vi "LVObject to JSON - No Data Member - Returns Type.vi"() -> ()   [LabVIEW 2017, in "Generic Object Serializer Tests.lvlib" / "Type Name Handling.lvlib"]
uses:
  Type Name Handling.lvlib
  No Data Member Subclass/No Data Member Subclass.lvclass
  Generic Object Serializer/Generic Object Serializer.lvclass
  Generic Object Serializer/Type Name Handling.ctl
  Generic Object Serializer/Generic Object Serializer.lvclass/Generic Object Serializer.ctl
  Generic Object Serializer/Write Type Name Handling.vi
  <vilib>/addons/_JKI Toolkits/Caraya/classes/Assert/Assert Equal Value_Variant.vi
  <vilib>/addons/_JKI Toolkits/Caraya/classes/Test/Test.lvclass
  <vilib>/addons/_JKI Toolkits/Caraya/classes/Assert/Assert.lvclass
panel:
  out "error out":errorcluster
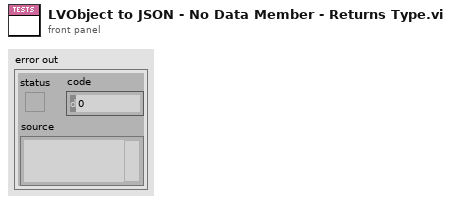
[diagram p1: front panel]
types:
  T1 = typedef "Generic Object Serializer.lvclass/Type Name Handling.ctl" = enum16{"None", "Inline"}
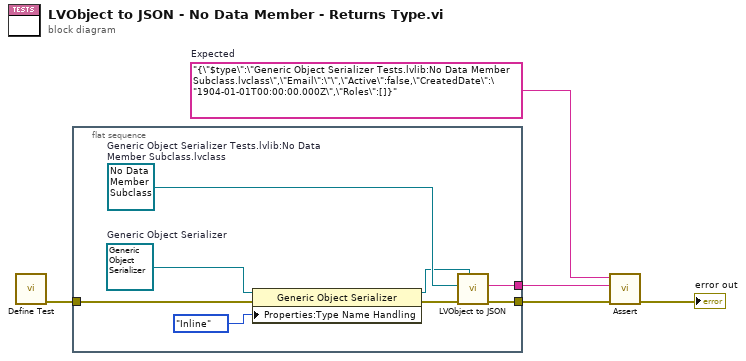
[diagram p0: block diagram]
diagram:
  w2 = "{\"$type\":\"Generic Object Serializer Tests.lvlib:No Data Member Subclass.lvclass\",\"Email\":\"\",\"Active\":false,\"CreatedDate\":\"1904-01-01T00:00:00.000Z\",\"Roles\":[]}"  # Expected
  n1 = call <vilib>:"Define Test.vi"() -> ("error out"=w5:errorcluster)  [unwired: 11 in]
  n2 = flat-sequence {
    tunnel: w5 -> [w7]
    tunnel: [w13] -> w4
    tunnel: [w11] -> w3
    frame #0 {
      w10 = refnum<class "Generic Object Serializer.lvclass"> refnum  # Generic Object Serializer
      w12 = refnum<class "No Data Member Subclass.lvclass"> refnum  # Generic Object Serializer Tests.lvlib:No Data Member Subclass.lvclass
      n3 = property class="Generic Object Serializer"(reference=w10, error in=w7, "Properties:Type Name Handling"=Type_Name_Handling."Inline" ("Type Name Handling")) -> (reference out=w9:refnum<class "Generic Object Serializer.lvclass">, error out=w6:errorcluster)
      n4 = call-dynamic "LVObject to JSON.vi"("LVClass Serializer"=w9, "error in (no error)"=w6, "Object"=w12) -> ("error out"=w13:errorcluster, "<JSON>Object"=w11:string)  [unwired: 7 in]
    }
  }
  n5 = call-poly <vilib>:"Assert.vi"("error in (no error)"=w4, "Y"=w3, "X"=w2) -> ("error out"=→"error out":errorcluster)  [unwired: 8 in]
